vi "InfoFileUpdate.vi"(8 "error in":errorcluster, 10 "File Paths":T1={"Local Save Path"=path "\\\\smbhome.uscs.susx.ac.uk\\cv222/Desktop/data", "Newton Save Path"=path "Z:/#Projects/Entanglement/data", "File Name"="test", "LocalSave"=TRUE}, 11 "info msg":string) -> (0 "error out":errorcluster)   [LabVIEW 2019]
uses:
  controls/FilePaths.ctl
  controls/GlobalExp.vi
  Global.lvlib
panel:
  in  "Cluster":cluster{"ExpNum":dbl, "ExpType":string} {"ExpNum" format="%_3f"}
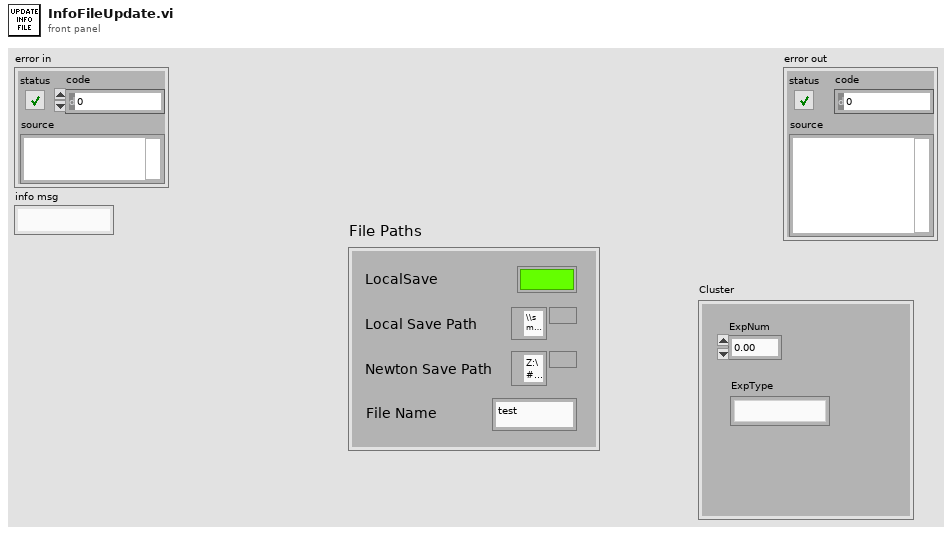
[diagram p1: front panel]
types:
  T1 = typedef "FilePaths.ctl" = cluster{"Local Save Path":path, "Newton Save Path":path, "File Name":string, "LocalSave":bool}
  T2 = enum16{"open", "replace", "create", "open or create", "replace or create", "replace or create with confirmation"}
  T3 = typedef "MasterExpControl.ctl" = cluster{"Main Steps":dbl, "Main Runs":dbl, "ExpStatus":enum16{"Innit", "Stop", "Idle", "MainRunning", "AuxRunning"}, "Main Current Step":dbl, "ExpNum":dbl, "NewData":bool, "date":string, "command":string, "Stop":bool, "Pause":bool, "Mathematica":string, "Main/Meta":bool, "UpdateMath":bool, "Camera":bool, "MetaExpOver":bool, "NextMetaExp":bool}
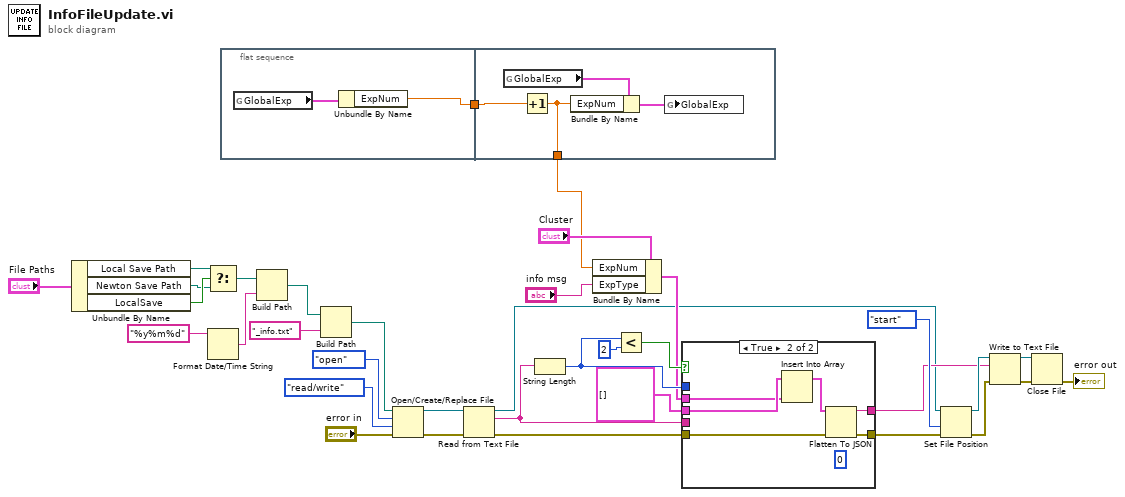
[diagram p0: block diagram]
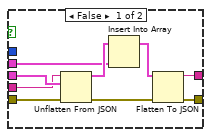
[diagram p2: hidden frame]
diagram:
  n1 = Unbundle By Name("File Paths") -> ("Local Save Path"=w32:path, "Newton Save Path"=w31:path, "LocalSave"=w33:bool)
  n2 = Select(t=w32, s=w33, f=w31) -> (s? t:f=w29:path)
  n3 = Format Date/Time String(time format string (%c)="%y%m%d") -> (date/time string=w30:string)  [unwired: 2 in]
  n4 = flat-sequence {
    tunnel: [w36] -> w2
    tunnel: w2 -> [w40]
    tunnel: [w38] -> w1
    frame #0 {
      n5 = global read "GlobalExp.vi" "GlobalExp"() -> (w37:T3)
      n6 = Unbundle By Name(w37) -> ("ExpNum"=w36:dbl)
    }
    frame #1 {
      n7 = global read "GlobalExp.vi" "GlobalExp"() -> (w39:T3)
      n8 = Increment(x=w40) -> (x+1=w38:dbl)
      n9 = Bundle By Name(cluster=w39, "ExpNum"=w38) -> (w41:T3)
      n10 = global write "GlobalExp.vi" "GlobalExp"(w41) -> ()
    }
  }
  n11 = Build Path(base path=w29, name or relative path=w30) -> (appended path=w27:path)
  n12 = Build Path(base path=w27, name or relative path="_info.txt") -> (appended path=w24:path)
  n13 = Open/Create/Replace File(file path (use dialog)=w24, error in="error in", operation (0:open)=T2."open", access (0:read/write)=enum16{"read/write", "read-only", "write-only"}."read/write") -> (refnum out=w25:refnum<file>, error out=w26:errorcluster)  [unwired: 2 in, 1 out]
  n14 = Read from Text File(file (use dialog)=w25, error in=w26) -> (refnum out=w4:refnum<file>, text=w18:string, error out=w16:errorcluster)  [unwired: 2 in, 1 out]
  n15 = String Length(string=w18) -> (length=w19:i32)
  n16 = Bundle By Name(cluster="Cluster", "ExpNum"=w1, "ExpType"="info msg") -> (w14:cluster{"ExpNum":dbl, "ExpType":string})
  n17 = Less?(x=w19, y=2) -> (x < y?=w21:bool)
  n18 = case shown="True" w21 {
    tunnel: w19 -> [_ _]
    tunnel: w18 -> [w47 _]
    tunnel: w16 -> [w50 w51]
    tunnel: cluster{"ExpNum":dbl, "ExpType":string}[] [] -> [w48 w56]
    tunnel: w14 -> [w46 w55]
    tunnel: [w44 w53] -> w5
    tunnel: [w43 w52] -> w6
    frame False {
      n19 = Unflatten From JSON(JSON string=w47, type and defaults=w48, error in (no error)=w50) -> (value=w49:cluster{"ExpNum":dbl, "ExpType":string}[], error out=w42:errorcluster)  [unwired: 4 in]
      n20 = Insert Into Array(array=w49, new element=w46) -> (w45:cluster{"ExpNum":dbl, "ExpType":string}[])  [unwired: 1 in]
      n21 = Flatten To JSON(anything=w45, error in (no error)=w42) -> (JSON string=w44:string, 11:w43:errorcluster)  [unwired: 1 in]
    }
    frame True {
      (unwired) i16 0 ("ExpNum")
      n22 = Insert Into Array(array=w56, new element=w55) -> (w54:cluster{"ExpNum":dbl, "ExpType":string}[])  [unwired: 1 in]
      n23 = Flatten To JSON(anything=w54, error in (no error)=w51) -> (JSON string=w53:string, 11:w52:errorcluster)  [unwired: 1 in]
    }
  }
  n24 = Set File Position(refnum=w4, from (0:start)=enum16{"start", "end", "current"}."start", error in=w6) -> (refnum out=w9:refnum<file>, error out=w8:errorcluster)  [unwired: 1 in]
  n25 = Write to Text File(file (use dialog)=w9, text=w5, error in=w8) -> (refnum out=w13:refnum<file>, error out=w12:errorcluster)  [unwired: 1 in, 1 out]
  n26 = Close File(refnum=w13, error in=w12) -> (error out=→"error out":errorcluster)  [unwired: 1 out]
